vi "Conn Status Global.vi"() -> ()   [LabVIEW 2012]
panel:
  out "Rdr Conn":bool
  in  "SteveTimeout LS":i32=2000 caption="LS"
  in  "SteveTimeout HS":i32=2000 caption="HS"
  out "Q Bcklg LS":i32
  out "Q Bcklg HS":i32
  out "LS Conn":bool
  out "HS Conn":bool
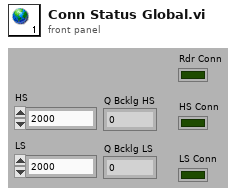
[diagram p1: front panel]
diagram:
